vi "calc ref.vi"(10 "dimension size":i32, 11 "Array":dbl[][][](array[numeric])) -> (1 "avg":dbl, 2 "ref even":i32, 3 "ref odd":i32)   [LabVIEW 2015]
panel:
  out "Waveform Graph 2":dbl[](graph)
  out "Waveform Graph":dbl[](graph)
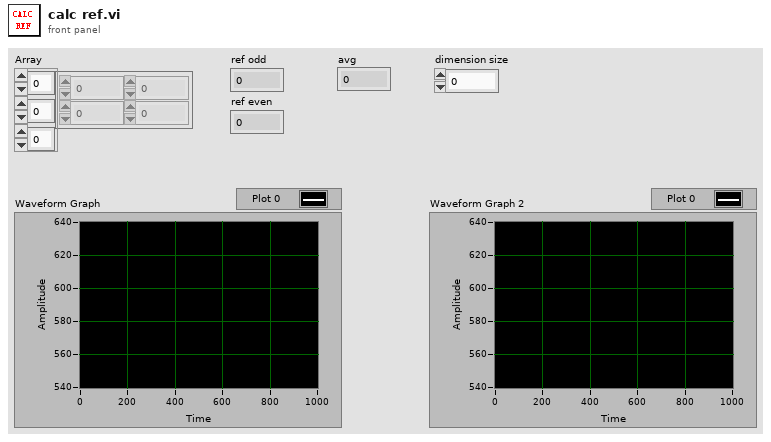
[diagram p1: front panel]
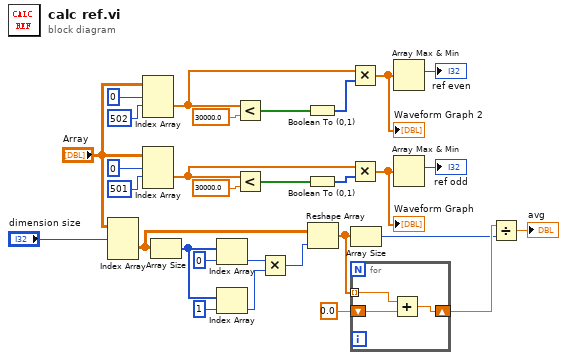
[diagram p0: block diagram]
diagram:
  n1 = Index Array(array="Array", index (dim 0)="dimension size") -> (element=w8:dbl[][])  [unwired: 2 in]
  n2 = Index Array(array="Array", index (dim 0)=0 ("index (page)"), index (dim 1)=502 ("disabled index (row)")) -> (element=w18:dbl[])  [unwired: 1 in]
  n3 = Index Array(array="Array", index (dim 0)=0 ("index (page)"), index (dim 1)=501 ("disabled index (row)")) -> (element=w23:dbl[])  [unwired: 1 in]
  n4 = Array Size(array=w8) -> (size(s)=w5:i32[])
  n5 = Index Array(array=w5, index=0) -> (element=w4:i32)
  n6 = Index Array(array=w5, index=1) -> (element=w3:i32)
  n7 = Less?(x=w18, y=30000.0) -> (x < y?=w20:bool[])
  n8 = Less?(x=w23, y=30000.0) -> (x < y?=w24:bool[])
  n9 = Multiply(x=w4, y=w3) -> (x*y=w2:i32)
  n10 = Boolean To (0,1)(Boolean=w20) -> (0, 1=w19:i16[])
  n11 = Boolean To (0,1)(Boolean=w24) -> (0, 1=w22:i16[])
  n12 = Reshape Array(w8, w2) -> (w1:dbl[])
  n13 = Multiply(x=w18, y=w19) -> (x*y=w16:dbl[])
  "Waveform Graph 2" <- w16
  n14 = Multiply(x=w23, y=w22) -> (x*y=w17:dbl[])
  "Waveform Graph" <- w17
  n15 = Array Size(array=w1) -> (size(s)=w11:i32)
  n16 = for {
    shift-right: [w32] -> w13
    shift-left: 0.0 -> [w33]
    tunnel: w1 -> [w31] mode=indexing
    n17 = Add(x=w31, y=w33) -> (x+y=w32:dbl)
  }
  n18 = Array Max & Min(array=w16) -> (max index (indices)=→"ref even":i32)  [unwired: 3 out]
  n19 = Array Max & Min(array=w17) -> (max index (indices)=→"ref odd":i32)  [unwired: 3 out]
  n20 = Divide(x=w13, y=w11) -> (x/y=→"avg":dbl)
